vi "Trajectory Box Monitor.vi"() -> ()   [LabVIEW 2017]
panel:
  in  "ID Status":string
  in  "?":enum32{"Option A", "Option B"}(tab)
  in  "Test Profile":T1(array[cluster])=[{"Ram Up Time"=10.0, "Hold Time"=5.0, "Ramp Down"=10.0, "Concentration Value"=25.0}, {"Ram Up Time"=15.0, "Hold Time"=10.0, "Ramp Down"=5.0, "Concentration Value"=35.0}, {"Ram Up Time"=0.0, "Hold Time"=0.0, "Ramp Down"=0.0, "Concentration Value"=0.0}]
  out "Profile Plotting":cluster{"X":dbl, "Y":dbl}[](graph)
  in  "Profile File Selection":u16(ring) items=["Test A", "Test B", "Test C"]
  in  "Iterations":dbl
  in  "Gas Selection":u16(ring) items=["Test A", "Test B", "Test C"]
  in  "Drive  2":string
  in  "Drive":string
  in  "IP Address":string
  in  "error in (no error)":errorcluster
  in  "Note":string
  in  "Tab- Main":enum32{"Settings", "Report", "Testscreen"}(tab)
  in  "Save Data Entry 2":bool
  in  "Tab Control Testscreen 4":enum32{"Channel Mapping", "Test Settings"}(tab)
  in  "Channel Mapping":T2(array[cluster])
  in  "Sampling Frequency (Hz)":string="Trajectory"
  in  "Wifi Name":string="Trajectory"
  out "Test Inactivity Time":dbl=30.0 format="%<%H:%M:%S>t"
  in  "Drive Path":path=path "D:/Trajectory Data"
  in  "cRIO IP Address":string="192.168.1.1"
  out "Test Time":dbl=1.0 format="%<%H:%M:%S>t"
  in  "Tab Control Testscreen 5":enum32{"Report", "Detailed Report"}(tab)
  out "Report Data":i32(listbox)
  in  "To Date & Time":timestamp format="%<%x>T"
  in  "From Date & Time":timestamp format="%<%x>T"
  in  "Test Stop Time :":string="12:59:05"
  in  "Tab Control Testscreen 6":enum32{"Data", "Histogram"}(tab)
  in  "Report Data 2":i32(listbox)
  out "XY Graph 3":cluster{i32, "Numeric":u16}[](graph)
  in  "ID Status :":string="00068OK"
  in  "ID :":string="Trajectory"
  in  "Angle :":string="Multi"
  in  "Flow :":string="Flow"
  in  "Material :":string="Cole"
  in  "Furnace :":string="G Furnace"
  in  "Test Start Time:":string="12:59:05"
  in  "Date :":string="02/07/2021"
  in  "Tab- Main 2":T3(tab)
  in  "Test details":T4={"Furnace"="Furnace A", "Material"="Coke", "Angle"="Multi Angle", "ID"="Trajectory 9", "Flowrate"="Flow", "Test Name"="Coke Burn", "Tested By"="Anirban"}
  in  "Save Data Entry":bool
  in  "Probe":bool[](array[boolean])
  in  "Probe 2":bool[](array[boolean])=[TRUE, FALSE, FALSE, FALSE, TRUE, FALSE, FALSE, FALSE, FALSE, FALSE, FALSE, FALSE, FALSE, FALSE, FALSE, FALSE, FALSE, FALSE, FALSE, FALSE, FALSE, FALSE, FALSE, FALSE, FALSE, FALSE, FALSE, FALSE, FALSE, FALSE, FALSE, FALSE, FALSE, FALSE, FALSE, FALSE, FALSE, FALSE, FALSE, FALSE, FALSE, FALSE, FALSE, FALSE, FALSE, FALSE, FALSE, FALSE, FALSE, FALSE, FALSE, FALSE, FALSE, FALSE, FALSE, FALSE, FALSE, FALSE, FALSE, FALSE]
  in  "Probe 3":bool[](array[boolean])=[TRUE, FALSE, FALSE, FALSE, TRUE, FALSE, FALSE, FALSE, FALSE, FALSE, FALSE, FALSE, FALSE, FALSE, FALSE, FALSE, FALSE, FALSE, FALSE, FALSE, FALSE, FALSE, FALSE, FALSE, FALSE, FALSE, FALSE, FALSE, FALSE, FALSE, FALSE, FALSE, FALSE, FALSE, FALSE, FALSE, FALSE, FALSE, FALSE, FALSE, FALSE, FALSE, FALSE, FALSE, FALSE, FALSE, FALSE, FALSE, FALSE, FALSE, FALSE, FALSE, FALSE, FALSE, FALSE, FALSE, FALSE, FALSE, FALSE, FALSE]
  out "Data Logging Path":path
  out "XY Graph":cluster{i32, "Numeric":u16}[](graph)
  in  "Setup":bool
  in  "Calibrations":bool
  in  "Disk Space Host":string="Trajectory 9"
  in  "Disk Space cRIO":string="Trajectory 9"
  in  "DataLog Duration":string="00:01:27"
  in  "Alarms":i32(listbox)
  out "Logging":bool=TRUE
  out "Logging 3":bool=TRUE
  in  "Stop Test":bool
  in  "Start Test":bool
  out "Message":string="Acquiring Data"
  in  "Test Screen":bool
  in  "Report":bool
  in  "Exit":bool
  in  "Settings":bool
  # "Trajectory Box Monitor System"
  # "03/07/2021 8:45:51"
  # "Test Setup Setting"
  # "1"
  # "5"
  # "10"
  # "15"
  # "20"
  # "21"
  # "25"
  # "30"
  # "40"
  # "35"
  # "41"
  # "45"
  # "50"
  # "55"
  # "60"
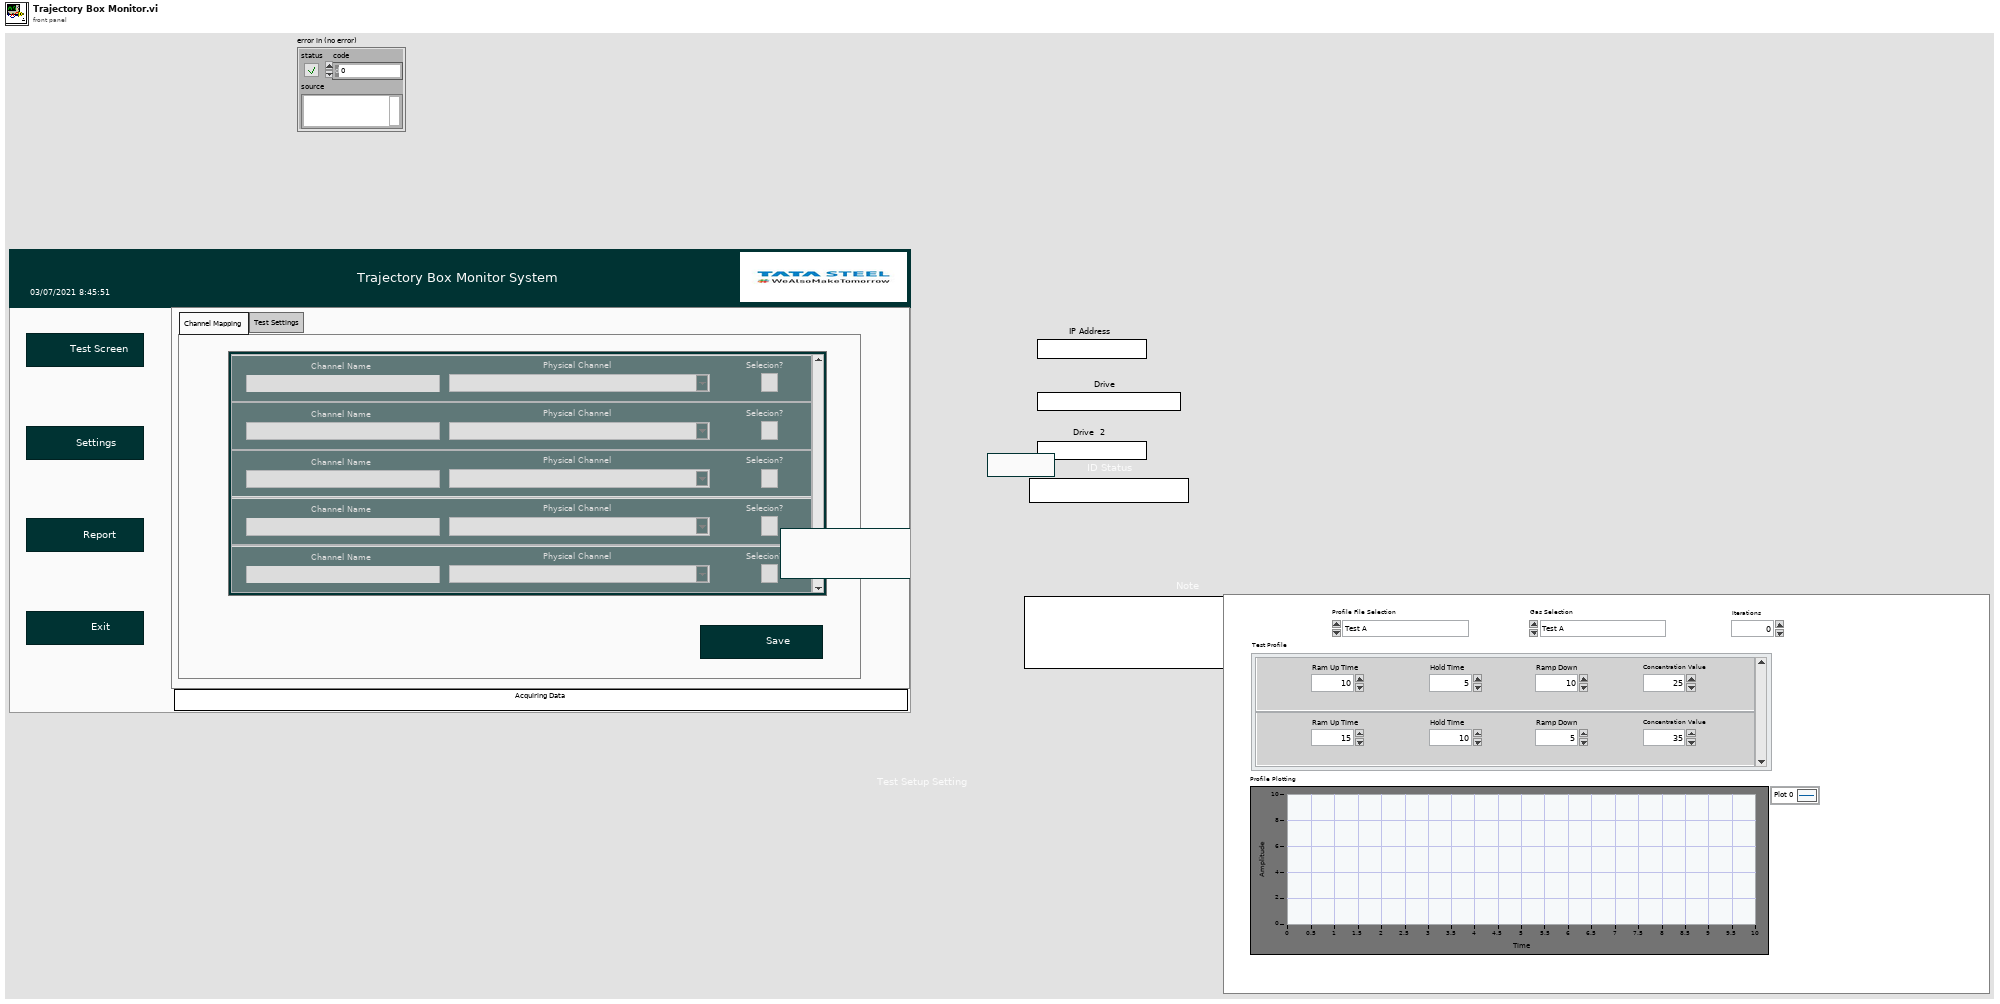
[diagram p1: front panel]
types:
  T1 = cluster{"Ram Up Time":dbl, "Hold Time":dbl, "Ramp Down":dbl, "Concentration Value":dbl}[]
  T2 = cluster{"Channel Name":string, " Physical Channel":tag, "Selecion?":bool}[]
  T3 = enum32{"Test Information", "Sensor Status", "Histogram", "Info", "Software Log"}
  T4 = cluster{"Furnace":string, "Material":string, "Angle":string, "ID":string, "Flowrate":string, "Test Name":string, "Tested By":string}
  T5 = cluster{"Channel Name":string, " Physical Channel":tag, "Selecion?":bool}
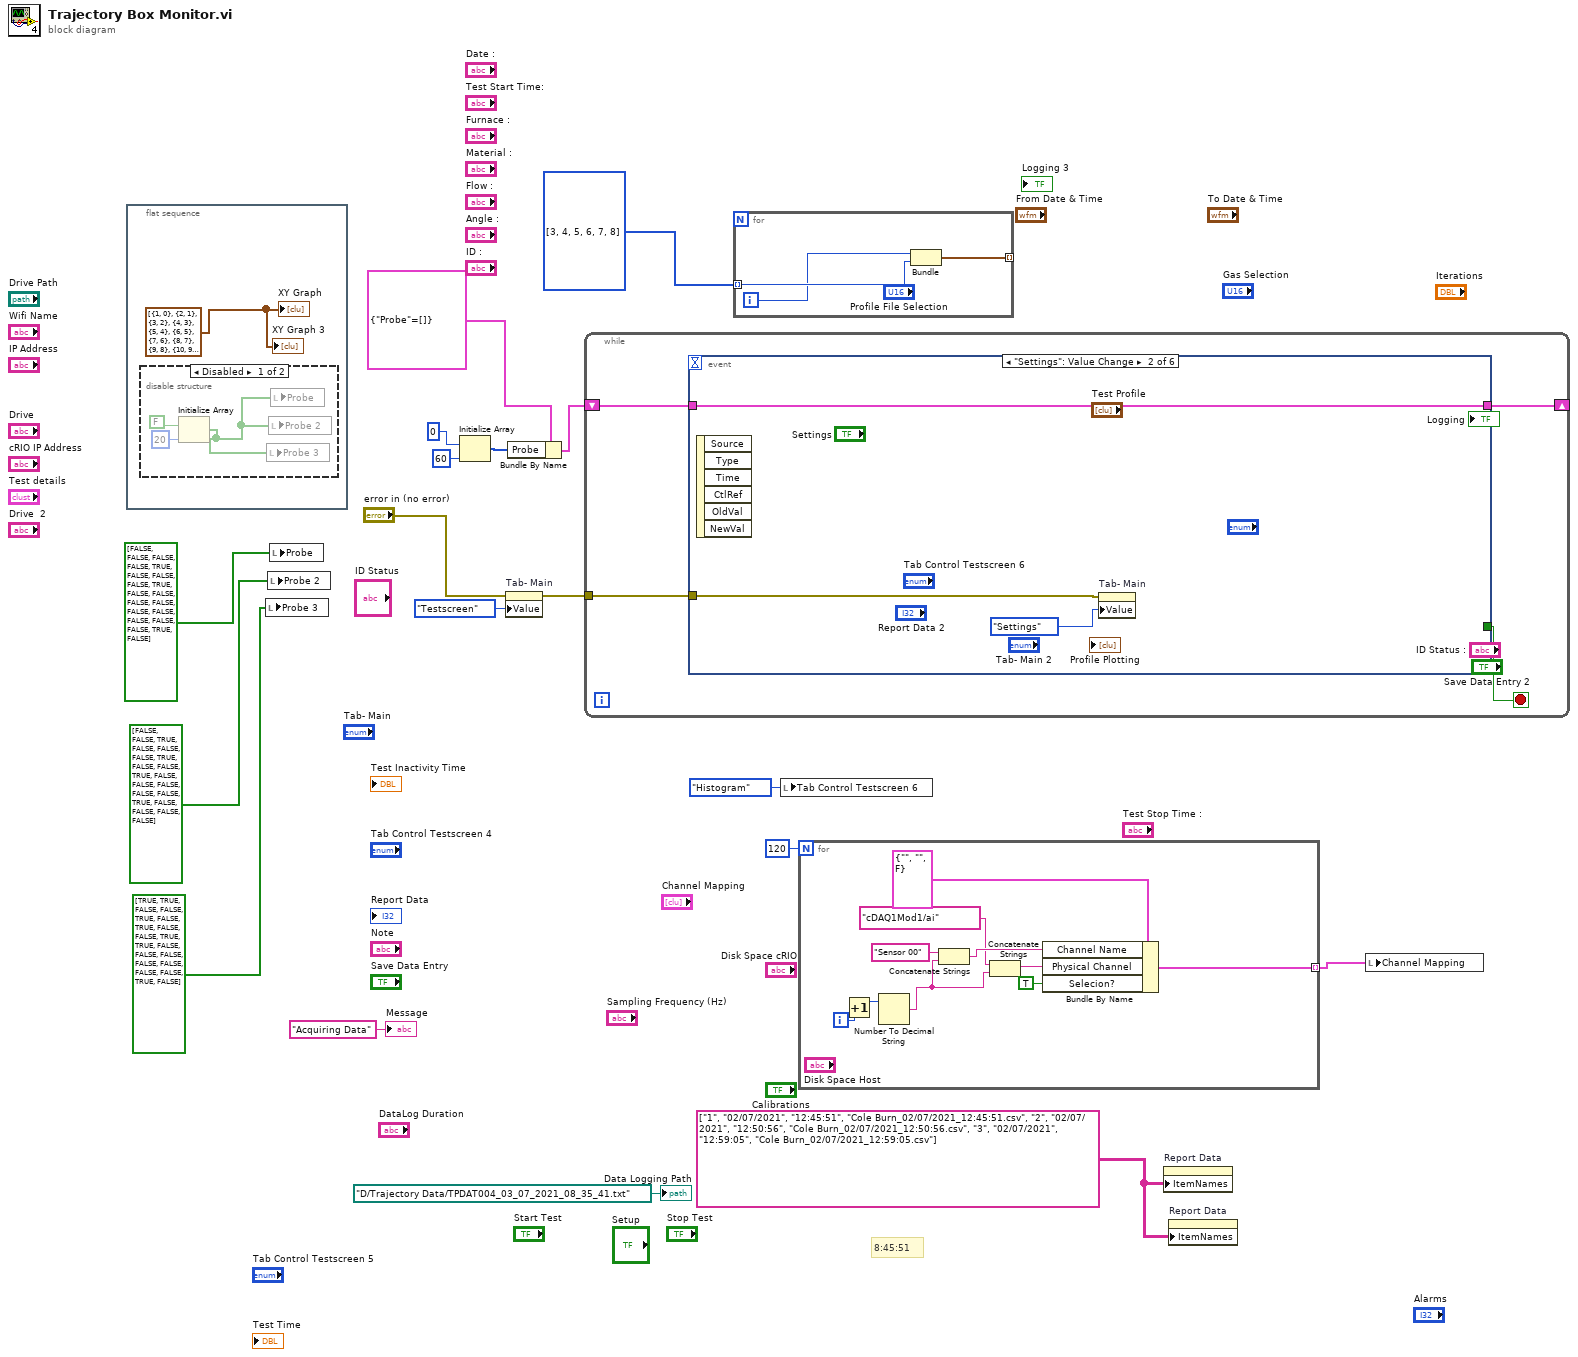
[diagram p0: block diagram]
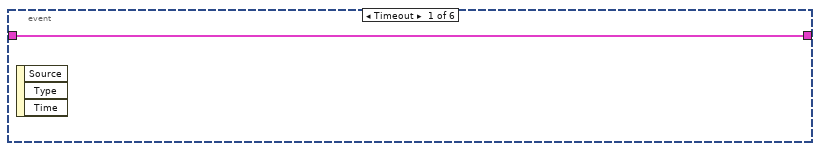
[diagram p3: hidden frame]
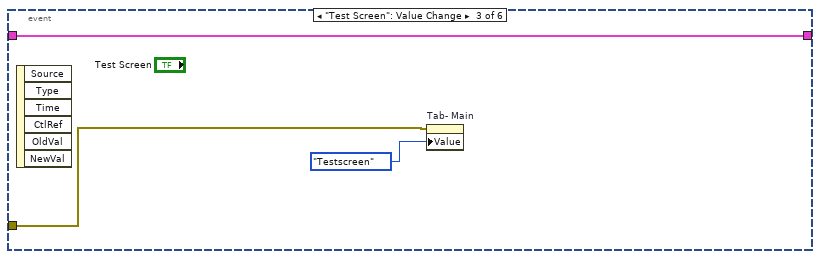
[diagram p4: hidden frame]
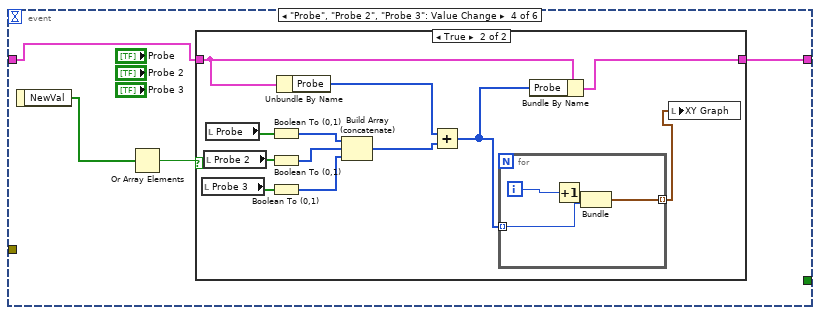
[diagram p5: hidden frame]
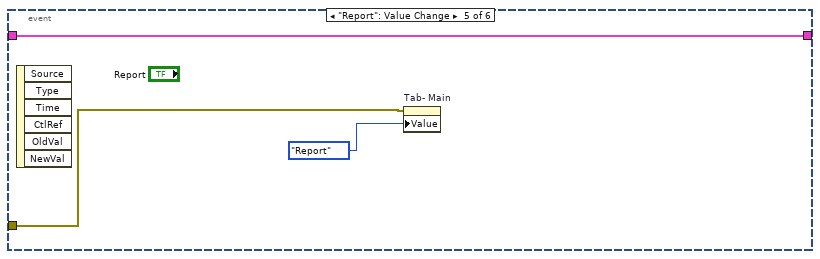
[diagram p7: hidden frame]
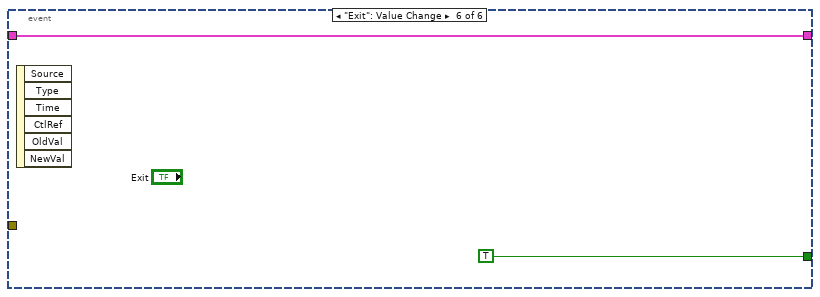
[diagram p8: hidden frame]
diagram:
  w1 = string[][] [["1", "02/07/2021", "12:45:51", "Cole Burn_02/07/2021_12:45:51.csv"], ["2", "02/07/2021", "12:50:56", "Cole Burn_02/07/2021_12:50:56.csv"], ["3", "02/07/2021", "12:59:05", "Cole Burn_02/07/2021_12:59:05.csv"]] ("Item Names")
  # "8:45:51"
  n1 = flat-sequence {
    frame #0 {
      w19 = cluster{i32, "Numeric":u16}[] [{1, "Numeric"=0}, {2, "Numeric"=1}, {3, "Numeric"=2}, {4, "Numeric"=3}, {5, "Numeric"=4}, {6, "Numeric"=5}, {7, "Numeric"=6}, {8, "Numeric"=7}, {9, "Numeric"=8}, {10, "Numeric"=9}, {11, "Numeric"=10}, {12, "Numeric"=11}, {13, "Numeric"=12}, {14, "Numeric"=13}, {15, "Numeric"=14}, {16, "Numeric"=15}, {17, "Numeric"=16}, {18, "Numeric"=17}, {19, "Numeric"=18}, {20, "Numeric"=19}, {21, "Numeric"=20}, {22, "Numeric"=21}, {23, "Numeric"=22}, {24, "Numeric"=23}, {25, "Numeric"=24}, {26, "Numeric"=25}, {27, "Numeric"=26}, {28, "Numeric"=27}, {29, "Numeric"=28}, {30, "Numeric"=29}, {30, "Numeric"=29}, {31, "Numeric"=28}, {32, "Numeric"=27}, {33, "Numeric"=26}, {34, "Numeric"=25}, {35, "Numeric"=24}, {36, "Numeric"=23}, {37, "Numeric"=22}, {38, "Numeric"=21}, {39, "Numeric"=20}, {40, "Numeric"=19}, {41, "Numeric"=18}, {42, "Numeric"=17}, {43, "Numeric"=16}, {44, "Numeric"=15}, {45, "Numeric"=14}, {46, "Numeric"=13}, {47, "Numeric"=12}, {48, "Numeric"=11}, {49, "Numeric"=10}, {50, "Numeric"=9}, {51, "Numeric"=8}, {52, "Numeric"=7}, {53, "Numeric"=6}, {54, "Numeric"=5}, {55, "Numeric"=4}, {56, "Numeric"=3}, {57, "Numeric"=2}, {58, "Numeric"=1}, {59, "Numeric"=0}] ("appended array 2")
      n2 = disable-structure shown="Disabled" {
        frame Disabled {
          n3 = Initialize Array(FALSE ("Boolean"), 20 ("dimension size")) -> (w20:bool[])
          n4 = local write "Probe 3"(w20) -> ()
          n5 = local write "Probe 2"(w20) -> ()
          n6 = local write "Probe"(w20) -> ()
        }
        frame Enabled {
        }
      }
      "XY Graph" <- w19
      "XY Graph 3" <- w19
    }
  }
  n7 = local write "Probe 3"(bool[] [TRUE, TRUE, FALSE, FALSE, TRUE, FALSE, TRUE, FALSE, FALSE, TRUE, TRUE, FALSE, FALSE, FALSE, FALSE, FALSE, FALSE, FALSE, TRUE, FALSE] ("Probe")) -> ()
  n8 = local write "Probe 2"(bool[] [FALSE, FALSE, TRUE, FALSE, FALSE, FALSE, TRUE, FALSE, FALSE, TRUE, FALSE, FALSE, FALSE, FALSE, FALSE, TRUE, FALSE, FALSE, FALSE, FALSE] ("Probe")) -> ()
  n9 = local write "Probe"(bool[] [FALSE, FALSE, FALSE, FALSE, TRUE, FALSE, FALSE, FALSE, TRUE, FALSE, FALSE, FALSE, FALSE, FALSE, FALSE, FALSE, FALSE, FALSE, TRUE, FALSE] ("Probe")) -> ()
  n10 = Initialize Array(0 ("Numeric"), 60 ("dimension size")) -> (w13:i32[])
  n11 = property on="Tab- Main" class="TabCtl (strict)"(error in="error in (no error)", "Value"=enum32{"Settings", "Report", "Testscreen"}."Testscreen" ("Tab- Main")) -> (error out=w17:errorcluster)  [unwired: 1 in, 1 out]
  n12 = Bundle By Name(cluster=cluster{"Probe":i32[]} {"Probe"=[]}, "Probe"=w13) -> (w11:cluster{"Probe":i32[]})
  n13 = while {
    tunnel: w17 -> [w25]
    shift-right: [w23] -> _
    shift-left: w11 -> [w24]
    stop <- w26 stop-if-true
    n14 = event shown="[1] \"Settings\": Value Change" {
      selector: _ -> [_ _ _ _ _ _]
      dyn-events: _ -> [_ _ _ _ _ _]
      timeout: _ -> [_ _ _ _ _ _]
      tunnel: [_ _ _ _ _ TRUE] -> w26
      tunnel: w25 -> [_ w30 w33 _ w57 _]
      tunnel: w24 -> [w27 w29 w32 w35 w56 w58]
      tunnel: [w27 w29 w32 w34 w56 w58] -> w23
      event Timeout {
        n15 = event-data() -> ()  [unwired: 1 in, 3 out]
      }
      event "Settings": Value Change {
        n16 = event-data() -> ()  [unwired: 1 in, 6 out]
        n17 = property on="Tab- Main" class="TabCtl (strict)"(error in=w30, "Value"=enum32{"Settings", "Report", "Testscreen"}."Settings" ("Tab- Main")) -> ()  [unwired: 1 in, 2 out]
      }
      event "Test Screen": Value Change {
        n18 = event-data() -> ()  [unwired: 1 in, 6 out]
        n19 = property on="Tab- Main" class="TabCtl (strict)"(error in=w33, "Value"=enum32{"Settings", "Report", "Testscreen"}."Testscreen" ("Tab- Main")) -> ()  [unwired: 1 in, 2 out]
      }
      event "Probe", "Probe 2", "Probe 3": Value Change {
        n20 = event-data() -> ("NewVal"=w37:bool[])  [unwired: 1 in]
        n21 = Or Array Elements(Boolean array=w37) -> (logical OR=w36:bool)
        n22 = case shown="True" w36 {
          tunnel: w35 -> [w38 w41]
          tunnel: [w38 w40] -> w34
          frame False {
          }
          frame True {
            n23 = local read "Probe 3"() -> (w48:bool[])
            n24 = local read "Probe 2"() -> (w49:bool[])
            n25 = local read "Probe"() -> (w50:bool[])
            n26 = Boolean To (0,1)(Boolean=w50) -> (0, 1=w47:i16[])
            n27 = Boolean To (0,1)(Boolean=w49) -> (0, 1=w46:i16[])
            n28 = Boolean To (0,1)(Boolean=w48) -> (0, 1=w45:i16[])
            n29 = Unbundle By Name(w41) -> ("Probe"=w44:i32[])
            n30 = Build Array (concatenate)(w47, w46, w45) -> (w43:i16[])
            n31 = Add(x=w44, y=w43) -> (x+y=w39:i32[])
            n32 = for {
              tunnel: [w54] -> w42 mode=indexing
              tunnel: w39 -> [w53] mode=indexing
              i -> [w52]
              n33 = Increment(x=w52) -> (x+1=w51:i32)
              n34 = Bundle(w51, w53) -> (w54:cluster{i32, i32})  [unwired: 1 in]
            }
            n35 = Bundle By Name(cluster=w41, "Probe"=w39) -> (w40:cluster{"Probe":i32[]})
            n36 = local write "XY Graph"(w42) -> ()
          }
        }
      }
      event "Report": Value Change {
        n37 = event-data() -> ()  [unwired: 1 in, 6 out]
        n38 = property on="Tab- Main" class="TabCtl (strict)"(error in=w57, "Value"=enum32{"Settings", "Report", "Testscreen"}."Report" ("Tab- Main")) -> ()  [unwired: 1 in, 2 out]
      }
      event "Exit": Value Change {
        n39 = event-data() -> ()  [unwired: 1 in, 6 out]
      }
    }
  }
  n40 = for {
    tunnel: [w62] -> _ mode=indexing
    tunnel: u16[] [3, 4, 5, 6, 7, 8] -> [w61] mode=indexing
    i -> [w60]
    n41 = Bundle(w60, "Numeric"=w61) -> (w62:cluster{i32, "Numeric":u16})  [unwired: 1 in]
  }
  n42 = local write "Tab Control Testscreen 6"(enum32{"Data", "Histogram"}."Histogram" ("Tab Control Testscreen 6")) -> ()
  n43 = for {
    N: 120 -> [_]
    tunnel: [w63] -> w3 mode=indexing
    i -> [w70]
    n44 = Increment(x=w70) -> (x+1=w66:i32)
    n45 = Number To Decimal String(number=w66) -> (decimal integer string=w67:string)  [unwired: 1 in]
    n46 = Concatenate Strings("Sensor 00" ("string"), w67) -> (w69:string)
    n47 = Concatenate Strings("cDAQ1Mod1/ai" ("string"), w67) -> (w65:string)
    n48 = Bundle By Name(cluster=T5 {"Channel Name"="", " Physical Channel"="", "Selecion?"=FALSE} ("Channel Mapping"), "Channel Name"=w69, "Physical Channel"=w65, "Selecion?"=TRUE) -> (w63:T5)
  }
  n49 = property on="Report Data" class="MCListbox (strict)"("ItemNames"=w1) -> ()  [unwired: 2 in, 2 out]
  n50 = property on="Report Data" class="MCListbox (strict)"("ItemNames"=w1) -> ()  [unwired: 2 in, 2 out]
  n51 = local write "Channel Mapping"(w3) -> ()
  "Message" <- "Acquiring Data" ("Message")
  "Data Logging Path" <- path "D:/Trajectory Data/TPDAT004_03_07_2021_08_35_41.txt" ("Data Logging Path")
